vi "Set Buffer and Get Channel Reading.vi"(8 "error in":errorcluster, 9 "Readings":waveform(dbl)[](array[waveform]), 10 "Channel Ident":string, 11 "BufferLastReadsWAV in":refnum<class "BufferLastReadsWAV.lvclass">) -> (0 "error out":errorcluster, 2 "Last Read":variant, 3 "BufferLastReadsWAV out":refnum<class "BufferLastReadsWAV.lvclass">)   [LabVIEW 2024, in "BufferLastReadsWAV.lvclass"]
uses:
  BufferLastReadsWAV.lvclass
  BufferLastReadsWAV.lvclass/BufferLastReadsWAV.ctl
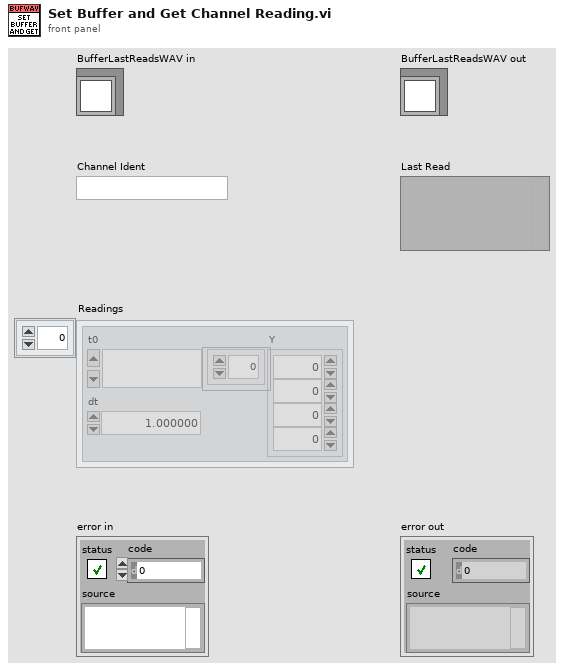
[diagram p1: front panel]
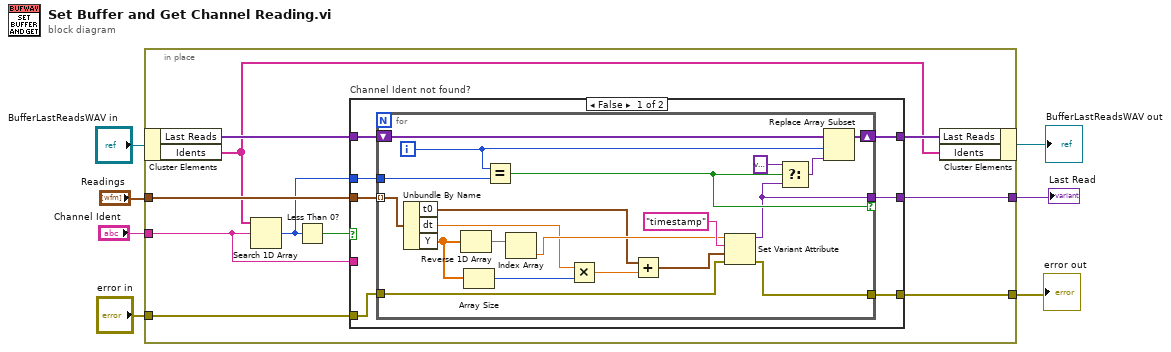
[diagram p0: block diagram]
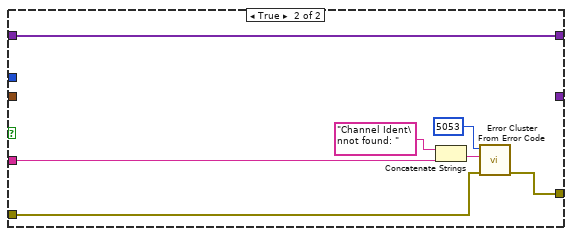
[diagram p2: hidden frame]
diagram:
  n1 = in-place {
    in-place-border: "Readings" -> [w17]
    in-place-border: "Channel Ident" -> [w9]
    in-place-border: "error in" -> [w11]
    in-place-border: [w10] -> w4
    in-place-border: [w8] -> w1
    n2 = in-place-cluster #1("BufferLastReadsWAV in") -> ("Last Reads"=w16:variant[], "Idents"=w13:string[])
    n3 = Search 1D Array(1D array=w13, element=w9) -> (index of element=w14:i32)  [unwired: 1 in]
    n4 = Less Than 0?(x=w14) -> (x < 0?=w12:bool)
    n5 = case "Channel Ident not found?" shown="False" w12 {
      tunnel: w17 -> [w24 _]
      tunnel: w16 -> [w23 w45]
      tunnel: [w22 w45] -> w15
      tunnel: w14 -> [w21 _]
      tunnel: w11 -> [w20 w48]
      tunnel: [w19 w47] -> w10
      tunnel: w9 -> [_ w46]
      tunnel: [w18 _] -> w8
      frame False {
        n6 = for {
          tunnel: [w34] -> w18 if=w44
          tunnel: w24 -> [w31] mode=indexing
          shift-right: [w39] -> w22
          shift-left: w23 -> [w42]
          tunnel: w21 -> [w38]
          tunnel: w20 -> [w36]
          tunnel: [w35] -> w19
          i -> [w41]
          n7 = Unbundle By Name(w31) -> ("t0"=w25:timestamp, "dt"=w27:dbl, "Y"=w30:dbl[])
          n8 = Reverse 1D Array(array=w30) -> (reversed array=w33:dbl[])
          n9 = Array Size(array=w30) -> (size(s)=w29:i32)
          n10 = Equal?(x=w41, y=w38) -> (x = y?=w44:bool)
          n11 = Index Array(array=w33) -> (element=w32:dbl)  [unwired: 1 in]
          n12 = Multiply(x=w27, y=w29) -> (x*y=w28:dbl)
          n13 = Add(x=w25, y=w28) -> (x+y=w26:timestamp)
          n14 = Set Variant Attribute(Variant=w32, name="timestamp", value=w26, error in=w36) -> (Variant out=w34:variant, error out=w35:errorcluster)  [unwired: 1 out]
          n15 = Select(t=variant, s=w44, f=w34) -> (s? t:f=w40:variant)
          n16 = Replace Array Subset(array=w42, new element=w40, index=w41) -> (w39:variant[])
        }
      }
      frame True {
        n17 = Concatenate Strings("Channel Ident\nnot found: " ("error message (\"\")"), w46) -> (w51:string)
        n18 = call <vilib>:"Error Cluster From Error Code.vi"("error in (no error)"=w48, "error message (\"\")"=w51, "error code (0)"=5053) -> ("error out"=w47:errorcluster)  [unwired: 6 in]
      }
    }
    n19 = in-place-cluster #1("Last Reads"=w15, "Idents"=w13) -> (→"BufferLastReadsWAV out":refnum<class "BufferLastReadsWAV.lvclass">)
  }
  "error out" <- w4
  "Last Read" <- w1
